vi "Button And Latch.vi"(0 "Swtich 2":bool, 1 "Latch 3":bool, 3 "Reset":bool, 5 "Swtich 3":bool, 7 "Latch 1":bool, 11 "Latch 2":bool, 12 "Stop":bool) -> (4 "Time(ms) 7":u32, 6 "Time(ms) 8":u32, 10 "Time(ms) 9":dbl, 14 "Time(ms)":u32)   [LabVIEW 2014]
doc: "Simulates mechanical action of a switch and a latch in differnt mechanical conditions."
panel:
  out "LED 6":bool
  out "Time(ms) 11":u32
  out "LED 5":bool
  out "Time(ms)":dbl
  out "LED 4":bool
  out "LED 3":bool
  out "LED 2":bool
  out "LED 1":bool
  in  "Switch 1":bool
  # "Button Mechanical Action Simulation"
  # "Displays total time for which the LED is ON."
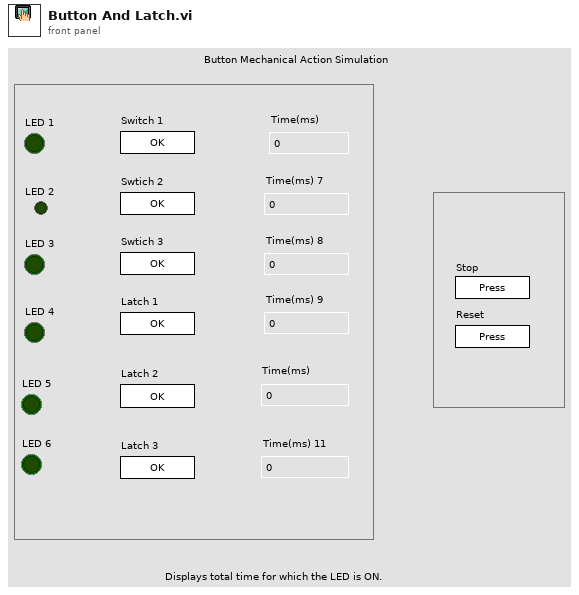
[diagram p1: front panel]
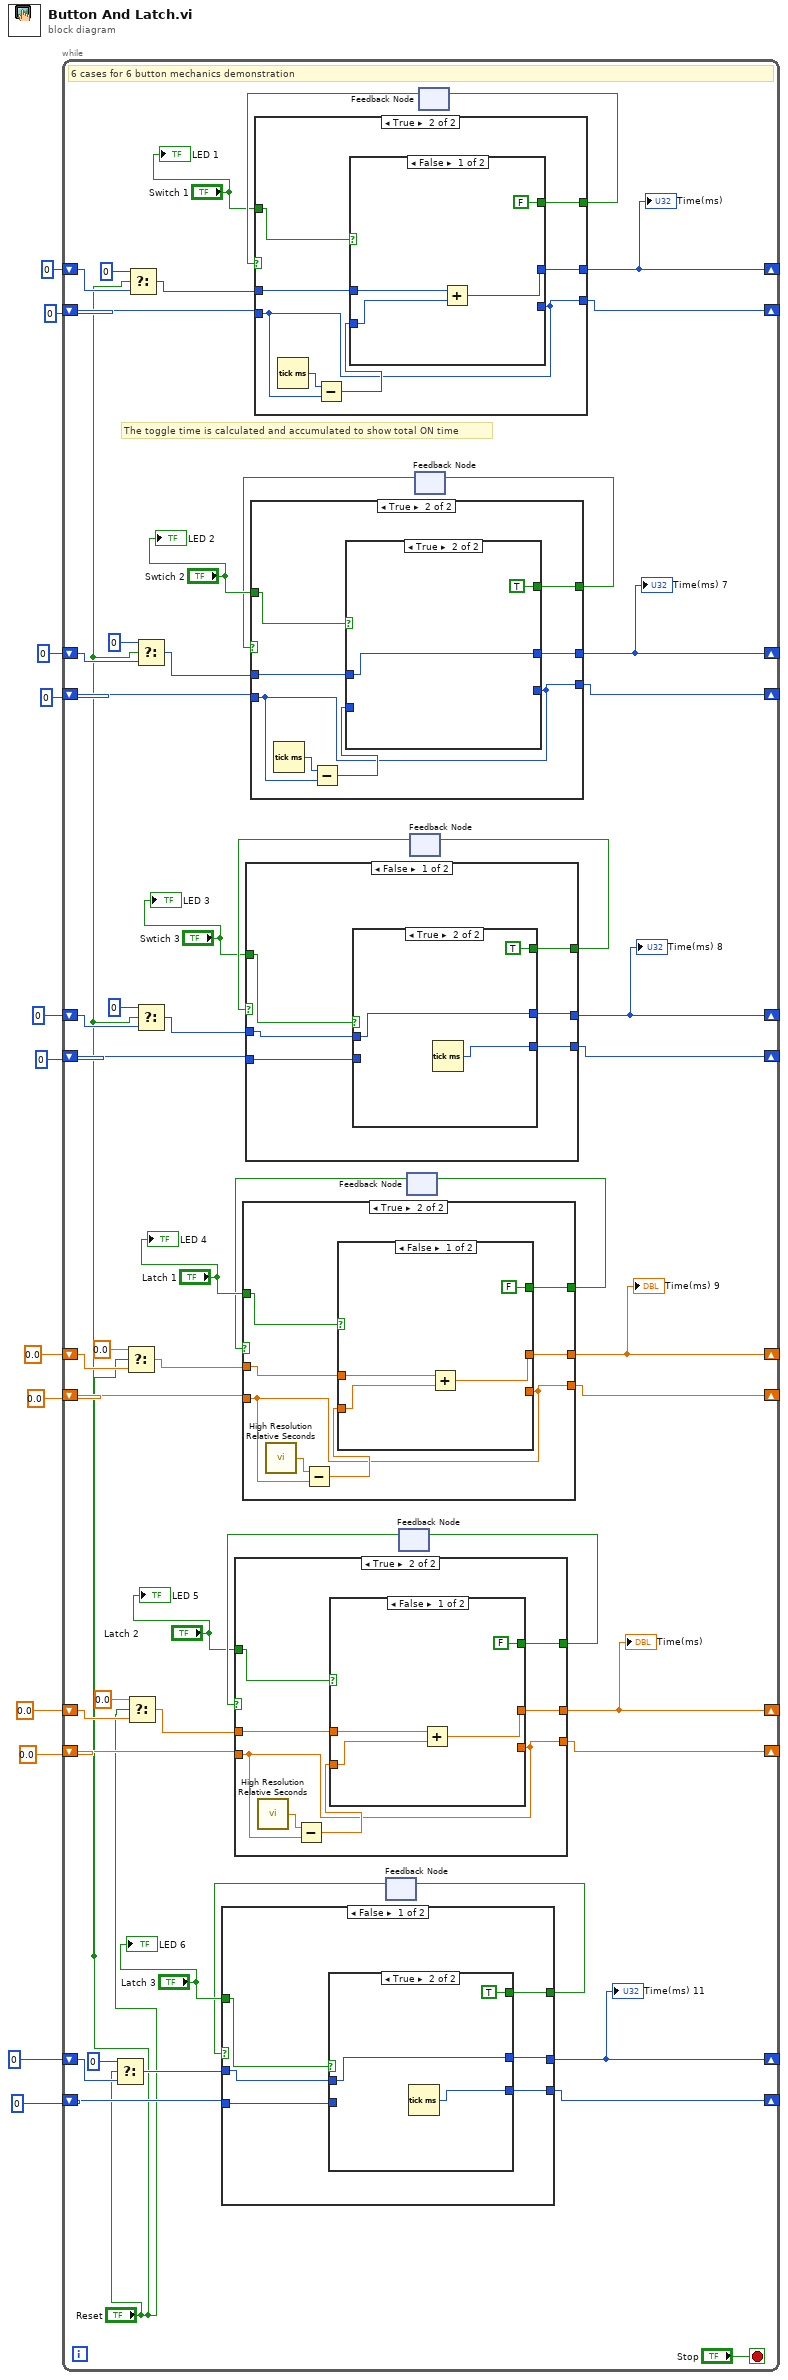
[diagram p0: block diagram]
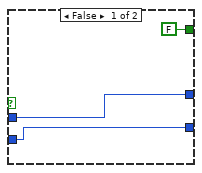
[diagram p2: hidden frame]
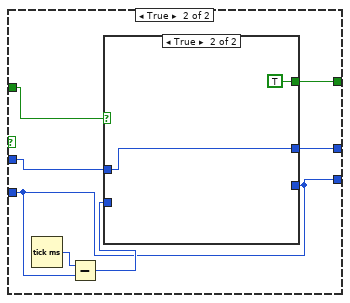
[diagram p3: hidden frame]
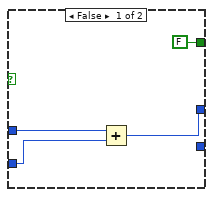
[diagram p4: hidden frame]
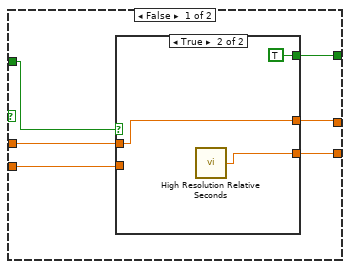
[diagram p5: hidden frame]
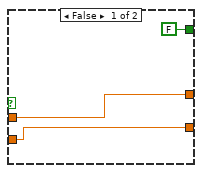
[diagram p6: hidden frame]
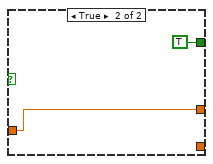
[diagram p7: hidden frame]
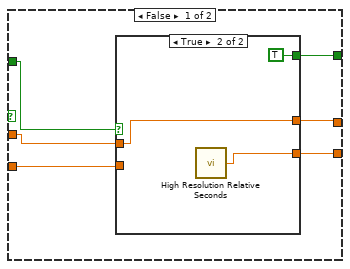
[diagram p8: hidden frame]
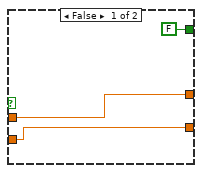
[diagram p9: hidden frame]
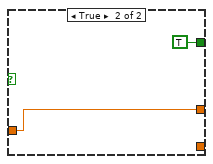
[diagram p10: hidden frame]
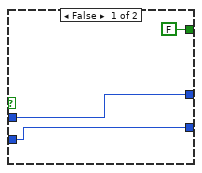
[diagram p11: hidden frame]
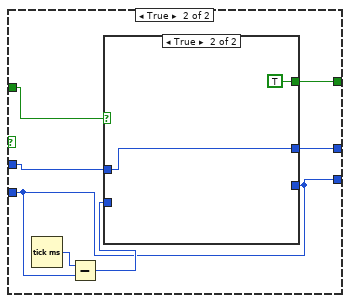
[diagram p12: hidden frame]
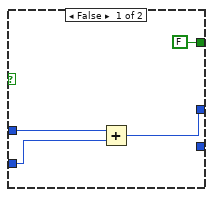
[diagram p13: hidden frame]
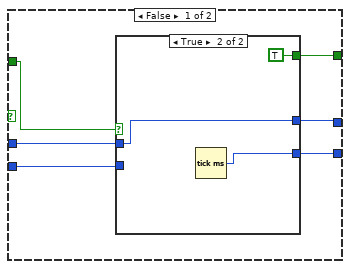
[diagram p14: hidden frame]
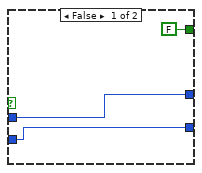
[diagram p15: hidden frame]
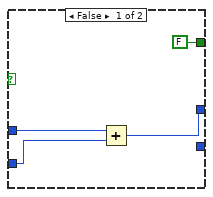
[diagram p16: hidden frame]
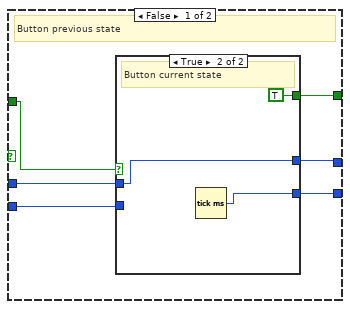
[diagram p17: hidden frame]
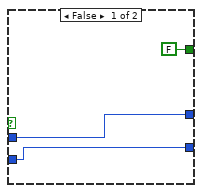
[diagram p18: hidden frame]
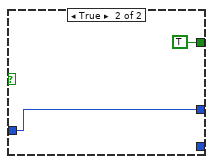
[diagram p19: hidden frame]
diagram:
  n1 = while {
    shift-right: [w68] -> _
    shift-left: u32 0 ("millisecond timer value") -> [w67]
    shift-right: [w64] -> _
    shift-left: u32 0 -> [w65]
    shift-right: [w56] -> _
    shift-left: u32 0 ("millisecond timer value") -> [w57]
    shift-right: [w59] -> _
    shift-left: u32 0 -> [w18]
    shift-right: [w55] -> _
    shift-left: u32 0 ("millisecond timer value") -> [w54]
    shift-right: [w52] -> _
    shift-left: u32 0 -> [w21]
    shift-right: [w44] -> _
    shift-left: 0.0 ("millisecond timer value") -> [w45]
    shift-right: [w47] -> _
    shift-left: 0.0 -> [w24]
    shift-right: [w43] -> _
    shift-left: 0.0 ("millisecond timer value") -> [w42]
    shift-right: [w40] -> _
    shift-left: 0.0 -> [w28]
    shift-right: [w31] -> _
    shift-left: u32 0 ("millisecond timer value") -> [w32]
    shift-right: [w34] -> _
    shift-left: u32 0 -> [w30]
    stop <- "Stop" stop-if-true
    # "The toggle time is calculated and accumulated to show total ON time"
    # "6 cases for 6 button mechanics demonstration"
    n2 = Select(t=u32 0, s="Reset", f=w30) -> (s? t:f=w27:u32)
    n3 = Select(t=0.0, s="Reset", f=w24) -> (s? t:f=w22:dbl)
    n4 = Select(t=0.0, s="Reset", f=w28) -> (s? t:f=w25:dbl)
    n5 = Select(t=u32 0, s="Reset", f=w65) -> (s? t:f=w14:u32)
    n6 = Select(t=u32 0, s="Reset", f=w18) -> (s? t:f=w16:u32)
    n7 = Select(t=u32 0, s="Reset", f=w21) -> (s? t:f=w19:u32)
    n8 = feedback #1() -> (w35:bool)  [unwired: 1 in]
    n9 = case shown="False" w35 {
      tunnel: [w74 w82] -> w31
      tunnel: w32 -> [w73 w82]
      tunnel: [w72 w84] -> w33
      tunnel: [w71 w85] -> w34
      tunnel: "Latch 3" -> [w70 w83]
      tunnel: w27 -> [w69 w81]
      frame False {
        n10 = case shown="True" w70 {
          tunnel: [w75 w80] -> w74
          tunnel: w73 -> [w75 _]
          tunnel: [FALSE TRUE] -> w72
          tunnel: w69 -> [w77 w78]
          tunnel: [w77 w78] -> w71
          frame False {
          }
          frame True {
            n11 = Tick Count (ms)() -> (millisecond timer value=w80:u32)
          }
        }
      }
      frame True {
        n12 = Tick Count (ms)() -> (millisecond timer value=w87:u32)
        n13 = Subtract(x=w87, y=w82) -> (x-y=w86:u32)
        n14 = case shown="True" w83 {
          tunnel: w86 -> [w91 _]
          tunnel: [w90 w92] -> w85
          tunnel: w81 -> [w89 w92]
          tunnel: [FALSE TRUE] -> w84
          tunnel: w82 -> [_ _]
          frame False {
            n15 = Add(x=w89, y=w91) -> (x+y=w90:u32)
          }
          frame True {
          }
        }
      }
    }
    "Time(ms) 11" <- w34
    n16 = feedback-in #1(w33) -> ()
    n17 = feedback #2() -> (w39:bool)  [unwired: 1 in]
    n18 = case shown="True" w39 {
      tunnel: [w99 w106] -> w43
      tunnel: w42 -> [w98 w106]
      tunnel: [w97 w108] -> w41
      tunnel: [w95 w110] -> w40
      tunnel: w25 -> [w96 w109]
      tunnel: "Latch 2" -> [w94 w107]
      frame False {
        n19 = case shown="True" w94 {
          tunnel: [w100 w105] -> w99
          tunnel: w98 -> [w100 _]
          tunnel: [FALSE TRUE] -> w97
          tunnel: w96 -> [w102 w103]
          tunnel: [w102 w103] -> w95
          frame False {
          }
          frame True {
            n20 = call <vilib>:"High Resolution Relative Seconds.vi"() -> ("relative seconds"=w105:dbl)
          }
        }
      }
      frame True {
        n21 = call <vilib>:"High Resolution Relative Seconds.vi"() -> ("relative seconds"=w112:dbl)
        n22 = Subtract(x=w112, y=w106) -> (x-y=w111:dbl)
        n23 = case shown="False" w107 {
          tunnel: w111 -> [w116 _]
          tunnel: [w115 w117] -> w110
          tunnel: w109 -> [w114 w117]
          tunnel: [FALSE TRUE] -> w108
          tunnel: w106 -> [_ _]
          frame False {
            n24 = Add(x=w114, y=w116) -> (x+y=w115:dbl)
          }
          frame True {
          }
        }
      }
    }
    "Time(ms)" <- w40
    n25 = feedback-in #2(w41) -> ()
    n26 = feedback #3() -> (w48:bool)  [unwired: 1 in]
    n27 = case shown="True" w48 {
      tunnel: [w124 w132] -> w44
      tunnel: w45 -> [w123 w132]
      tunnel: [w122 w134] -> w46
      tunnel: [w121 w135] -> w47
      tunnel: "Latch 1" -> [w120 w133]
      tunnel: w22 -> [w119 w131]
      frame False {
        n28 = case shown="True" w120 {
          tunnel: [w125 w130] -> w124
          tunnel: w123 -> [w125 _]
          tunnel: [FALSE TRUE] -> w122
          tunnel: w119 -> [w127 w128]
          tunnel: [w127 w128] -> w121
          frame False {
          }
          frame True {
            n29 = call <vilib>:"High Resolution Relative Seconds.vi"() -> ("relative seconds"=w130:dbl)
          }
        }
      }
      frame True {
        n30 = call <vilib>:"High Resolution Relative Seconds.vi"() -> ("relative seconds"=w137:dbl)
        n31 = Subtract(x=w137, y=w132) -> (x-y=w136:dbl)
        n32 = case shown="False" w133 {
          tunnel: w136 -> [w141 _]
          tunnel: [w140 w142] -> w135
          tunnel: w131 -> [w138 w142]
          tunnel: [FALSE TRUE] -> w134
          tunnel: w132 -> [_ _]
          frame False {
            n33 = Add(x=w138, y=w141) -> (x+y=w140:dbl)
          }
          frame True {
          }
        }
      }
    }
    "Time(ms) 9" <- w47
    n34 = feedback-in #3(w46) -> ()
    n35 = feedback #4() -> (w51:bool)  [unwired: 1 in]
    n36 = case shown="False" w51 {
      tunnel: [w149 w157] -> w55
      tunnel: w54 -> [w148 w157]
      tunnel: [w147 w159] -> w53
      tunnel: [w146 w160] -> w52
      tunnel: "Swtich 3" -> [w145 w158]
      tunnel: w19 -> [w144 w156]
      frame False {
        n37 = case shown="True" w145 {
          tunnel: [w150 w155] -> w149
          tunnel: w148 -> [w150 _]
          tunnel: [FALSE TRUE] -> w147
          tunnel: w144 -> [w152 w153]
          tunnel: [w152 w153] -> w146
          frame False {
          }
          frame True {
            n38 = Tick Count (ms)() -> (millisecond timer value=w155:u32)
          }
        }
      }
      frame True {
        n39 = Tick Count (ms)() -> (millisecond timer value=w162:u32)
        n40 = Subtract(x=w162, y=w157) -> (x-y=w161:u32)
        n41 = case shown="True" w158 {
          tunnel: w161 -> [w166 _]
          tunnel: [w165 w167] -> w160
          tunnel: w156 -> [w164 w167]
          tunnel: [FALSE TRUE] -> w159
          tunnel: w157 -> [_ _]
          frame False {
            n42 = Add(x=w164, y=w166) -> (x+y=w165:u32)
          }
          frame True {
          }
        }
      }
    }
    "Time(ms) 8" <- w52
    n43 = feedback-in #4(w53) -> ()
    n44 = feedback #5() -> (w60:bool)  [unwired: 1 in]
    n45 = case shown="True" w60 {
      tunnel: [w174 w181] -> w56
      tunnel: w57 -> [w173 w181]
      tunnel: [w172 w183] -> w58
      tunnel: [w170 w185] -> w59
      tunnel: w16 -> [w171 w184]
      tunnel: "Swtich 2" -> [w169 w182]
      frame False {
        n46 = case shown="True" w169 {
          tunnel: [w175 w180] -> w174
          tunnel: w173 -> [w175 _]
          tunnel: [FALSE TRUE] -> w172
          tunnel: w171 -> [w177 w178]
          tunnel: [w177 w178] -> w170
          frame False {
          }
          frame True {
            n47 = Tick Count (ms)() -> (millisecond timer value=w180:u32)
          }
        }
      }
      frame True {
        n48 = Tick Count (ms)() -> (millisecond timer value=w187:u32)
        n49 = Subtract(x=w187, y=w181) -> (x-y=w186:u32)
        n50 = case shown="True" w182 {
          tunnel: w186 -> [w191 _]
          tunnel: [w190 w192] -> w185
          tunnel: w184 -> [w189 w192]
          tunnel: [FALSE TRUE] -> w183
          tunnel: w181 -> [_ _]
          frame False {
            n51 = Add(x=w189, y=w191) -> (x+y=w190:u32)
          }
          frame True {
          }
        }
      }
    }
    "Time(ms) 7" <- w59
    n52 = feedback-in #5(w58) -> ()
    n53 = feedback #6() -> (w63:bool)  [unwired: 1 in]
    n54 = case shown="True" w63 {
      tunnel: [w199 w206] -> w68
      tunnel: w67 -> [w198 w206]
      tunnel: [w197 w208] -> w66
      tunnel: [w195 w210] -> w64
      tunnel: w14 -> [w196 w209]
      tunnel: "Switch 1" -> [w194 w207]
      frame False {
        # "Button previous state"
        n55 = case shown="True" w194 {
          tunnel: [w200 w205] -> w199
          tunnel: w198 -> [w200 _]
          tunnel: [FALSE TRUE] -> w197
          tunnel: w196 -> [w202 w203]
          tunnel: [w202 w203] -> w195
          frame False {
          }
          frame True {
            # "Button current state"
            n56 = Tick Count (ms)() -> (millisecond timer value=w205:u32)
          }
        }
      }
      frame True {
        n57 = Tick Count (ms)() -> (millisecond timer value=w212:u32)
        n58 = Subtract(x=w212, y=w206) -> (x-y=w211:u32)
        n59 = case shown="False" w207 {
          tunnel: w211 -> [w216 _]
          tunnel: [w215 w217] -> w210
          tunnel: w209 -> [w214 w217]
          tunnel: [FALSE TRUE] -> w208
          tunnel: w206 -> [_ _]
          frame False {
            n60 = Add(x=w214, y=w216) -> (x+y=w215:u32)
          }
          frame True {
          }
        }
      }
    }
    "Time(ms)" <- w64
    n61 = feedback-in #6(w66) -> ()
    "LED 1" <- "Switch 1"
    "LED 2" <- "Swtich 2"
    "LED 3" <- "Swtich 3"
    "LED 4" <- "Latch 1"
    "LED 5" <- "Latch 2"
    "LED 6" <- "Latch 3"
  }
